vi "avgvi.vi"(11 "image in":sgl[][](array[numeric])) -> (3 "image out":sgl[][](array[numeric]))   [LabVIEW 2012]
uses:
  GFG/GFGnumericGet.vi
  GFG/GFG library.lvlib
panel:
  in  "avg":sgl[][][](array[numeric])
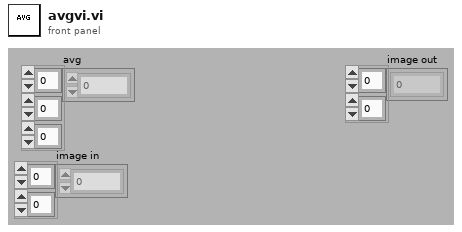
[diagram p1: front panel]
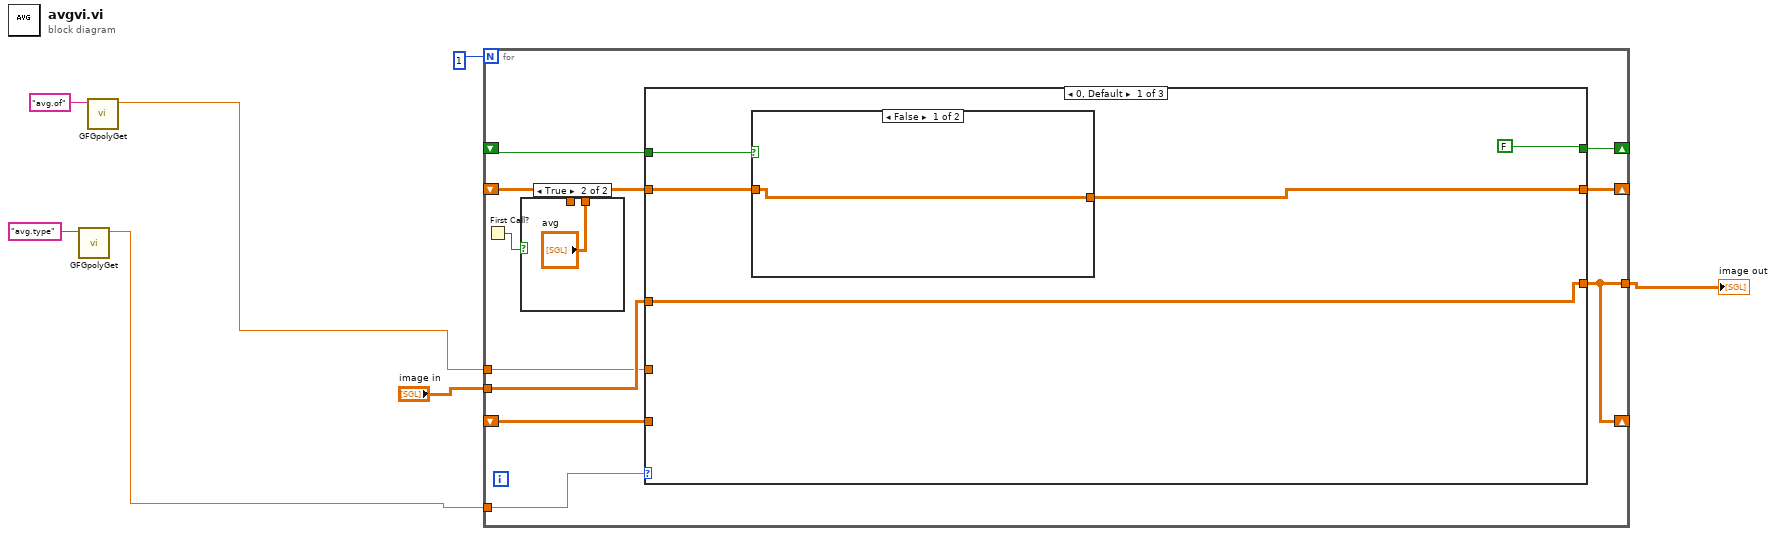
[diagram p0: block diagram]
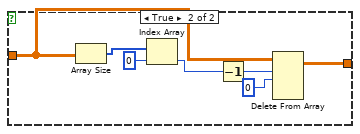
[diagram p2: hidden frame]
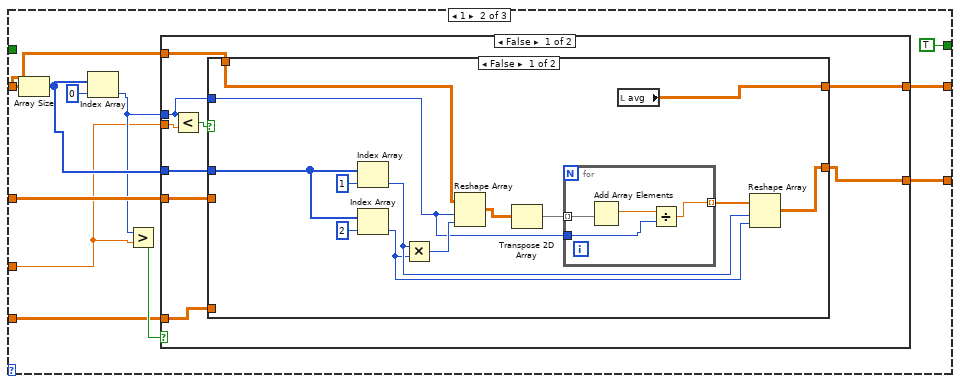
[diagram p3: hidden frame]
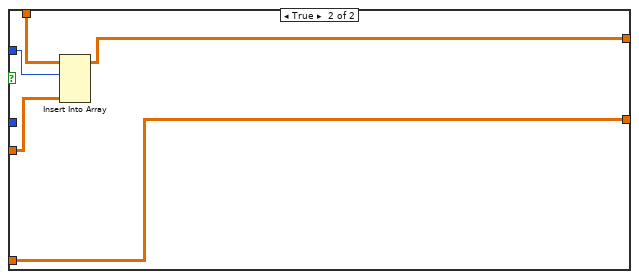
[diagram p4: hidden frame]
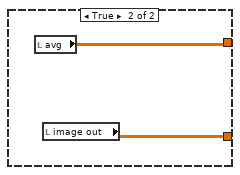
[diagram p5: hidden frame]
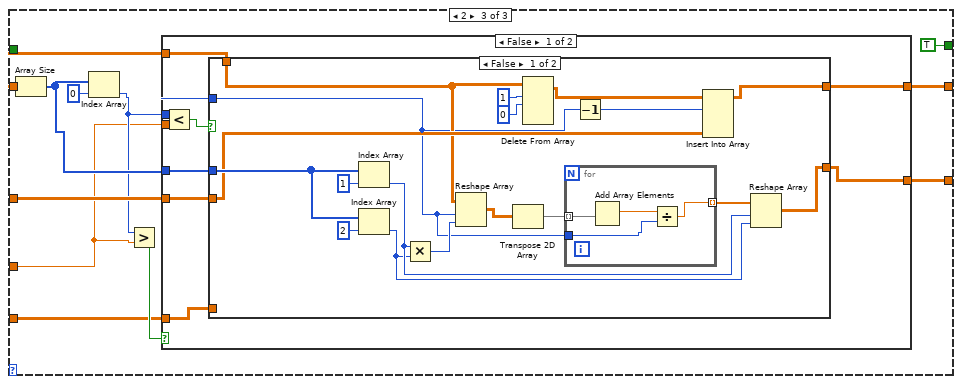
[diagram p6: hidden frame]
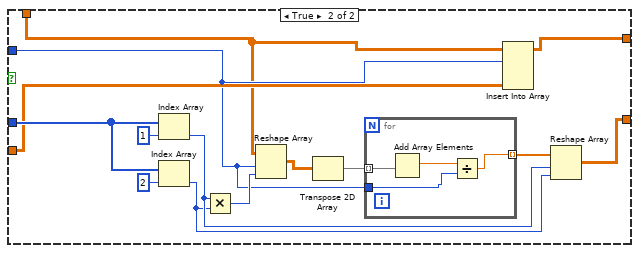
[diagram p7: hidden frame]
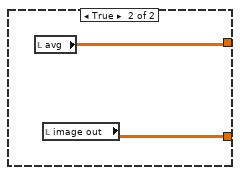
[diagram p8: hidden frame]
diagram:
  n1 = call-poly "GFGpolyGet.vi"("Variable Name in"="avg.type") -> ("Numeric"=w1:dbl)  [unwired: 9 in, 1 out]
  n2 = call-poly "GFGpolyGet.vi"("Variable Name in"="avg.of") -> ("Numeric"=w2:dbl)  [unwired: 9 in, 1 out]
  n3 = for {
    N: 1 -> [_]
    tunnel: "image in" -> [w18]
    shift-right: [w17] -> _
    shift-left: _ -> [w14]
    tunnel: [w11] -> w5
    tunnel: w1 -> [w13]
    tunnel: w2 -> [w12]
    shift-right: [w11] -> _
    shift-left: _ -> [w10]
    shift-right: [w8] -> _
    shift-left: _ -> [w9]
    n4 = First Call?() -> (First Call?: T/F=w15:bool)
    n5 = case shown="True" w15 {
      tunnel: [w138 "avg"] -> w16
      tunnel: w14 -> [w138 _]
      frame False {
      }
      frame True {
      }
    }
    n6 = case shown="0, Default" w13 {
      tunnel: w18 -> [w23 w41 w85]
      tunnel: [w21 w40 w84] -> w17
      tunnel: w16 -> [w22 w38 w82]
      tunnel: [w23 w37 w81] -> w11
      tunnel: w12 -> [_ w34 w78]
      tunnel: w10 -> [_ w33 w77]
      tunnel: w9 -> [w20 _ _]
      tunnel: [FALSE TRUE TRUE] -> w8
      frame 0, Default {
        n7 = case shown="False" w20 {
          tunnel: w22 -> [w24 w31]
          tunnel: [w24 w30] -> w21
          frame False {
          }
          frame True {
            n8 = Array Size(array=w31) -> (size(s)=w28:i32[])
            n9 = Index Array(array=w28, index=0) -> (element=w27:i32)
            n10 = Decrement(x=w27) -> (x-1=w26:i32)
            n11 = Delete From Array(array=w31, length=w26, index (dim 0)=0 ("index (page)")) -> (array with subset deleted=w30:sgl[][][])  [unwired: 2 in, 1 out]
          }
        }
      }
      frame 1 {
        n12 = Array Size(array=w38) -> (size(s)=w39:i32[])
        n13 = Index Array(array=w39, index=0) -> (element=w36:i32)
        n14 = Greater?(x=w36, y=w34) -> (0:w35:bool)
        n15 = case shown="False" w35 {
          tunnel: w34 -> [w51 _]
          tunnel: w41 -> [w50 _]
          tunnel: w36 -> [w49 _]
          tunnel: [w48 w74] -> w40
          tunnel: w39 -> [w46 _]
          tunnel: w38 -> [w45 _]
          tunnel: [w44 w75] -> w37
          tunnel: w33 -> [w43 _]
          frame False {
            n16 = Less?(x=w49, y=w51) -> (x < y?=w47:bool)
            n17 = case shown="False" w47 {
              tunnel: w50 -> [_ w71]
              tunnel: w49 -> [w53 w73]
              tunnel: [w52 w70] -> w48
              tunnel: w45 -> [w54 w72]
              tunnel: [w55 w69] -> w44
              tunnel: w46 -> [w63 _]
              tunnel: w43 -> [_ w69]
              frame False {
                n18 = Index Array(array=w63, index=1) -> (element=w57:i32)
                n19 = Index Array(array=w63, index=2) -> (element=w56:i32)
                n20 = Multiply(x=w57, y=w56) -> (x*y=w61:i32)
                n21 = Reshape Array(w54, w53, w61) -> (w60:sgl[][])
                n22 = Transpose 2D Array(2D array=w60) -> (transposed array=w59:sgl[][])
                n23 = for {
                  tunnel: w59 -> [w68] mode=indexing
                  tunnel: w53 -> [w67]
                  tunnel: [w65] -> w58 mode=indexing
                  n24 = Add Array Elements(numeric array=w68) -> (sum=w66:sgl)
                  n25 = Divide(x=w66, y=w67) -> (x/y=w65:sgl)
                }
                n26 = local read "avg"() -> (w52:sgl[][][])
                n27 = Reshape Array(w58, w57, w56) -> (w55:sgl[][])
              }
              frame True {
                n28 = Insert Into Array(array=w72, index (dim 0)=w73, new element=w71) -> (w70:sgl[][][])  [unwired: 2 in]
              }
            }
          }
          frame True {
            n29 = local read "avg"() -> (w74:sgl[][][])
            n30 = local read "image out"() -> (w75:sgl[][])
          }
        }
      }
      frame 2 {
        n31 = Array Size(array=w82) -> (size(s)=w83:i32[])
        n32 = Index Array(array=w83, index=0) -> (element=w80:i32)
        n33 = Greater?(x=w80, y=w78) -> (0:w79:bool)
        n34 = case shown="False" w79 {
          tunnel: w78 -> [w95 _]
          tunnel: w85 -> [w94 _]
          tunnel: w80 -> [w93 _]
          tunnel: [w92 w136] -> w84
          tunnel: w83 -> [w90 _]
          tunnel: w82 -> [w89 _]
          tunnel: [w88 w137] -> w81
          tunnel: w77 -> [w87 _]
          frame False {
            n35 = Less?(x=w93, y=w95) -> (x < y?=w91:bool)
            n36 = case shown="False" w91 {
              tunnel: w94 -> [w103 w121]
              tunnel: w93 -> [w98 w119]
              tunnel: [w96 w120] -> w92
              tunnel: w89 -> [w102 w118]
              tunnel: [w104 w122] -> w88
              tunnel: w90 -> [w112 w130]
              tunnel: w87 -> [_ _]
              frame False {
                n37 = Index Array(array=w112, index=1) -> (element=w106:i32)
                n38 = Index Array(array=w112, index=2) -> (element=w105:i32)
                n39 = Multiply(x=w106, y=w105) -> (x*y=w110:i32)
                n40 = Reshape Array(w102, w98, w110) -> (w109:sgl[][])
                n41 = Transpose 2D Array(2D array=w109) -> (transposed array=w108:sgl[][])
                n42 = Delete From Array(array=w102, length=1, index (dim 0)=0 ("index (page)")) -> (array with subset deleted=w101:sgl[][][])  [unwired: 2 in, 1 out]
                n43 = for {
                  tunnel: w108 -> [w117] mode=indexing
                  tunnel: w98 -> [w116]
                  tunnel: [w114] -> w107 mode=indexing
                  n44 = Add Array Elements(numeric array=w117) -> (sum=w115:sgl)
                  n45 = Divide(x=w115, y=w116) -> (x/y=w114:sgl)
                }
                n46 = Decrement(x=w98) -> (x-1=w97:i32)
                n47 = Insert Into Array(array=w101, index (dim 0)=w97, new element=w103) -> (w96:sgl[][][])  [unwired: 2 in]
                n48 = Reshape Array(w107, w106, w105) -> (w104:sgl[][])
              }
              frame True {
                n49 = Index Array(array=w130, index=1) -> (element=w124:i32)
                n50 = Index Array(array=w130, index=2) -> (element=w123:i32)
                n51 = Multiply(x=w124, y=w123) -> (x*y=w128:i32)
                n52 = Reshape Array(w118, w119, w128) -> (w127:sgl[][])
                n53 = Transpose 2D Array(2D array=w127) -> (transposed array=w126:sgl[][])
                n54 = for {
                  tunnel: w126 -> [w135] mode=indexing
                  tunnel: w119 -> [w134]
                  tunnel: [w132] -> w125 mode=indexing
                  n55 = Add Array Elements(numeric array=w135) -> (sum=w133:sgl)
                  n56 = Divide(x=w133, y=w134) -> (x/y=w132:sgl)
                }
                n57 = Insert Into Array(array=w118, index (dim 0)=w119, new element=w121) -> (w120:sgl[][][])  [unwired: 2 in]
                n58 = Reshape Array(w125, w124, w123) -> (w122:sgl[][])
              }
            }
          }
          frame True {
            n59 = local read "avg"() -> (w136:sgl[][][])
            n60 = local read "image out"() -> (w137:sgl[][])
          }
        }
      }
    }
  }
  "image out" <- w5
